vi "Write textColor.vi"(8 "error in (no error)":errorcluster, 10 "textColor":u32(colorbox), 11 "TextDecoration in":refnum<class "TextDecoration.lvclass">) -> (0 "error out":errorcluster, 3 "TextDecoration out":refnum<class "TextDecoration.lvclass">)   [LabVIEW 2023, in "TLC_Scripto.lvlib" / "TextDecoration.lvclass"]
uses:
  TextDecoration.lvclass
  Read textDecorationRef.vi
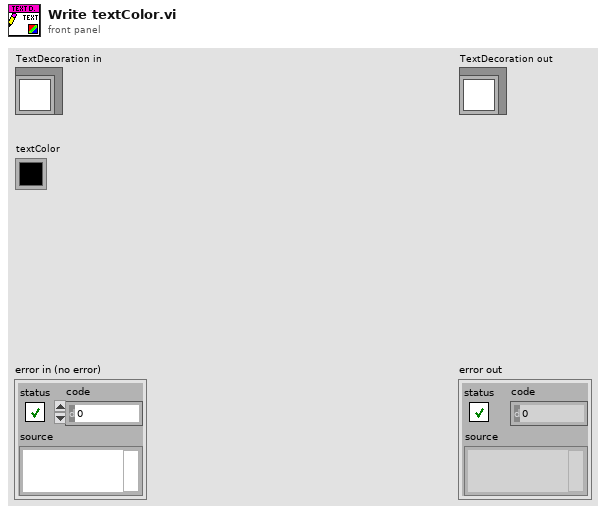
[diagram p1: front panel]
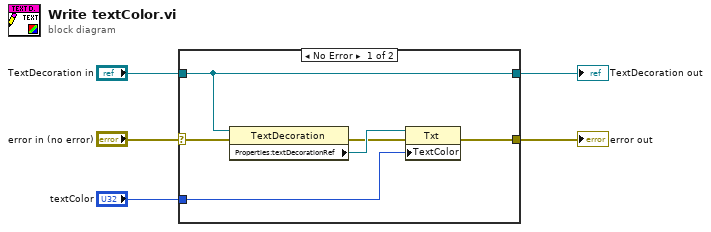
[diagram p0: block diagram]
diagram:
  n1 = case shown="No Error" "error in (no error)" {
    selector: "error in (no error)" -> [w9 w12]
    tunnel: [w8 w12] -> w4
    tunnel: [w7 w13] -> w2
    tunnel: "TextDecoration in" -> [w7 w13]
    tunnel: "textColor" -> [w6 _]
    frame No Error {
      n2 = property class="TextDecoration"(reference=w7, error in=w9) -> (error out=w10:errorcluster, "Properties:textDecorationRef"=w11:refnum<vi>)  [unwired: 1 out]
      n3 = property class="Txt"(reference=w11, error in=w10, "TextColor"=w6) -> (error out=w8:errorcluster)  [unwired: 1 out]
    }
    frame Error {
    }
  }
  "error out" <- w4
  "TextDecoration out" <- w2
